vi "Main (Host).vi"() -> ()   [LabVIEW 2014]
panel:
  in  "Subtract":bool
  in  "Add":bool
  out "Equals":dbl
  in  "B":dbl
  in  "A":dbl
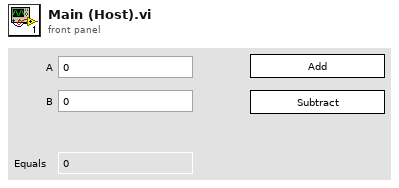
[diagram p1: front panel]
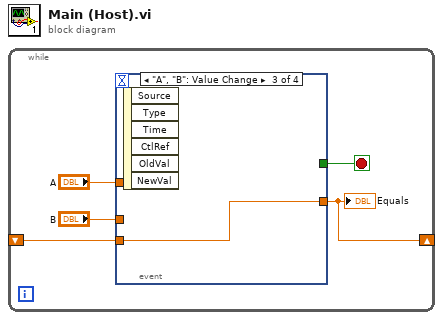
[diagram p0: block diagram]
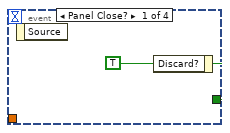
[diagram p2: hidden frame]
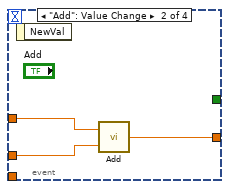
[diagram p3: hidden frame]
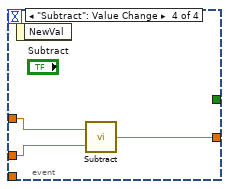
[diagram p4: hidden frame]
diagram:
  n1 = while {
    shift-right: [w2] -> _
    shift-left: _ -> [w1]
    stop <- w5 stop-if-true
    n2 = event shown="[2] \"A\", \"B\": Value Change" {
      selector: _ -> [_ _ _ _]
      dyn-events: _ -> [_ _ _ _]
      timeout: _ -> [_ _ _ _]
      tunnel: [w6 _ _ _] -> w5
      tunnel: "A" -> [_ w9 _ w13]
      tunnel: "B" -> [_ w8 _ w12]
      tunnel: [_ w7 w10 w11] -> w2
      tunnel: w1 -> [_ _ w10 _]
      event Panel Close? {
        w6 = TRUE ("Discard?")
        n3 = event-data() -> ()  [unwired: 1 in, 1 out]
        n4 = event-data("Discard?"=w6) -> ()  [unwired: 1 in, 1 out]
      }
      event "Add": Value Change {
        n5 = event-data() -> ()  [unwired: 1 in, 1 out]
        n6 = call "Add.vi"("B"=w8, "A"=w9) -> ("Sum"=w7:dbl)
      }
      event "A", "B": Value Change {
        n7 = event-data() -> ()  [unwired: 1 in, 6 out]
      }
      event "Subtract": Value Change {
        n8 = event-data() -> ()  [unwired: 1 in, 1 out]
        n9 = call "Subtract.vi"("B"=w12, "A"=w13) -> ("Sum"=w11:dbl)
      }
    }
    "Equals" <- w2
  }
